vi "ControlFuente.vi"(0 "DC OK 3":bool) -> (1 "DC OK 2":bool, 2 "DC OK":string, 3 "Boolean":bool)   [LabVIEW 2015]
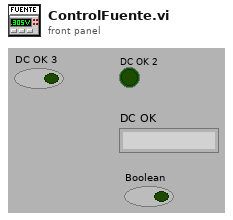
[diagram p1: front panel]
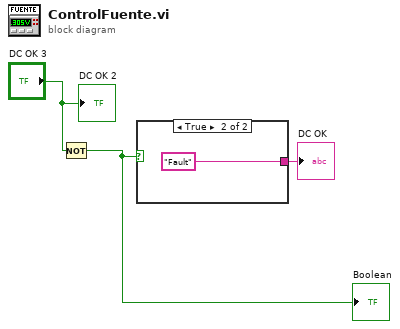
[diagram p0: block diagram]
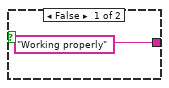
[diagram p2: hidden frame]
diagram:
  n1 = Not(x="DC OK 3") -> (.not. x?=w3:bool)
  "Boolean" <- w3
  n2 = case shown="True" w3 {
    tunnel: ["Working properly" "Fault"] -> w2
    frame False {
    }
    frame True {
    }
  }
  "DC OK" <- w2
  "DC OK 2" <- "DC OK 3"
